vi "ICM Select Channel Values.vi"(10 "Enabled":bool[](array[boolean]), 11 "Channel Values":dbl[](array[numeric])) -> (3 "Enabled Values":dbl[](array[numeric]))   [LabVIEW 2018]
doc: "ICM Select Channel Values.vi\n\nThis VI returns the values of the Channels that have been enabled in the configuration.\n\nInstrument Communication Module Version 1.0\nSeptember, 2017 Original Code Consulting David Thomson\n www.originalcode.com"
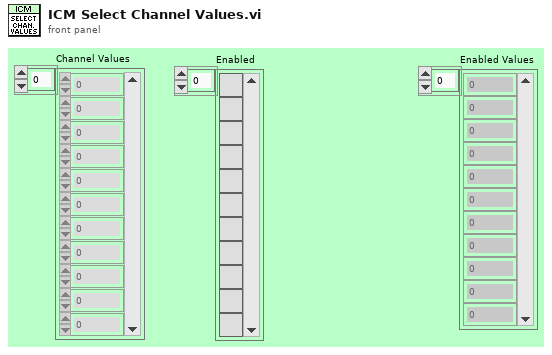
[diagram p1: front panel]
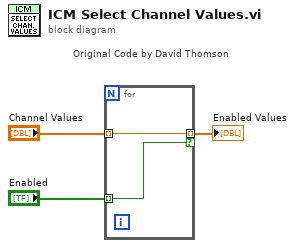
[diagram p0: block diagram]
diagram:
  n1 = for "Original Code by David Thomson" {
    tunnel: [w5] -> w1 mode=indexing if=w4
    tunnel: "Channel Values" -> [w5] mode=indexing
    tunnel: "Enabled" -> [w4] mode=indexing
  }
  "Enabled Values" <- w1
